vi "Task five.vi"() -> ()   [LabVIEW 2025]
uses:
  <vilib>/httpClient/POSTBuffer.vi
  <vilib>/httpClient/LabVIEWHTTPClient.lvlib
panel:
  in  "User Input":string
  in  "?":bool
  in  "Select correct word":string(combo)
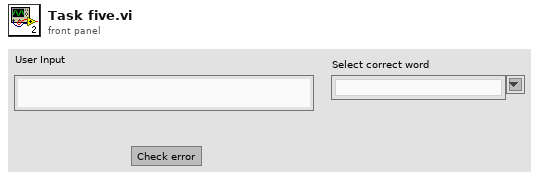
[diagram p1: front panel]
types:
  T1 = cluster{"matches":cluster{"offset":i32, "length":i32, "message":string, "replacements":cluster{"value":string}[]}[]}
  T2 = typedef "LabVIEWHTTPClient.lvlib/ClientHandle.ctl" = refnum<k1>
  T3 = cluster{"offset":i32, "length":i32, "message":string, "replacements":cluster{"value":string}[]}[]
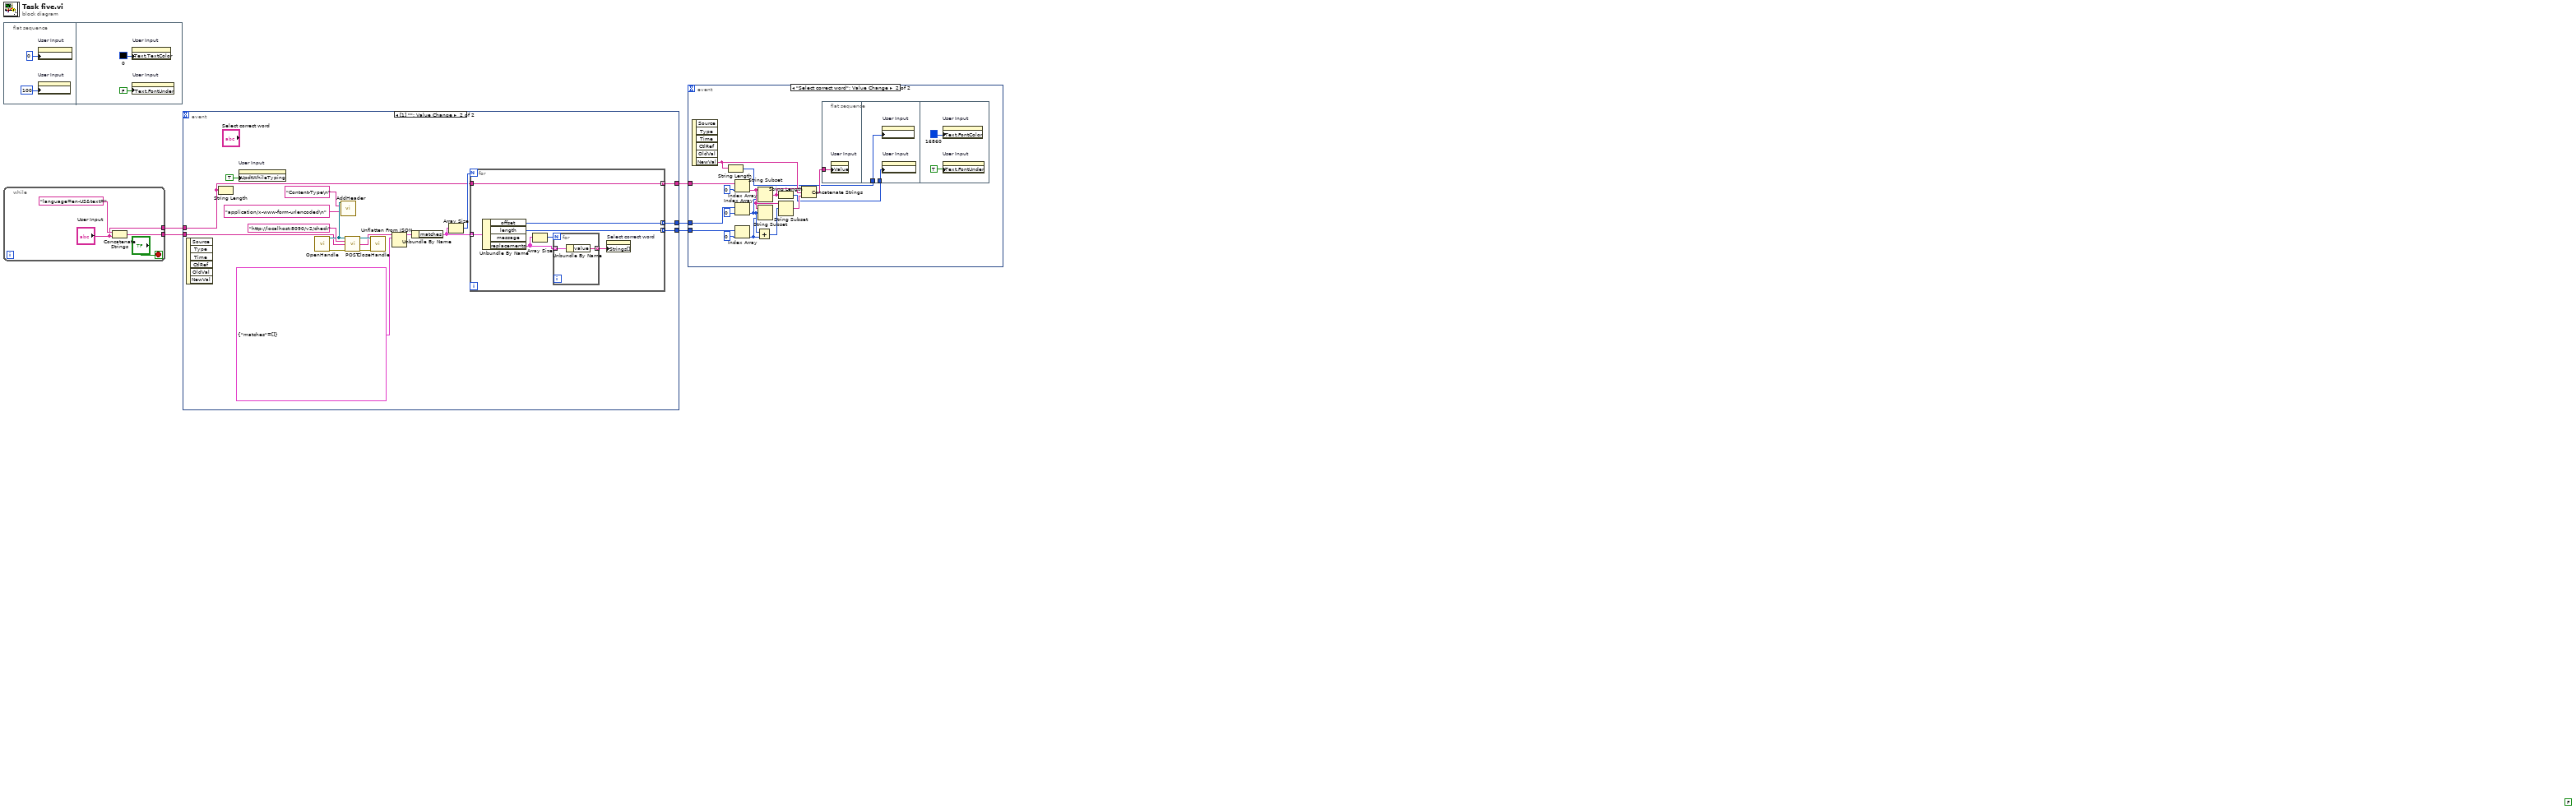
[diagram p0: block diagram]
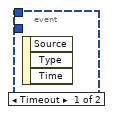
[diagram p2: hidden frame]
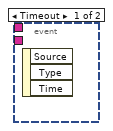
[diagram p3: hidden frame]
diagram:
  (unwired) FALSE
  n1 = flat-sequence {
    frame #0 {
      n2 = property on="User Input" class="Str"("Text.Selection Start"=0) -> ()  [unwired: 2 in, 2 out]
      n3 = property on="User Input" class="Str"("Text.Selection End"=100) -> ()  [unwired: 2 in, 2 out]
    }
    frame #1 {
      n4 = property on="User Input" class="Str"("Text.TextColor"=u32 0 ("Text.Font:Color")) -> ()  [unwired: 2 in, 2 out]
      n5 = property on="User Input" class="Str"("Text.FontUnder"=FALSE) -> ()  [unwired: 2 in, 2 out]
    }
  }
  n6 = while {
    tunnel: [w12] -> w2
    tunnel: ["User Input"] -> w1
    stop <- "?" stop-if-true
    n7 = Concatenate Strings("language=en-US&text=", "User Input") -> (w12:string)
  }
  n8 = event shown="[1] \"\": Value Change" {
    selector: _ -> [_ _]
    dyn-events: _ -> [_ _]
    timeout: _ -> [_ _]
    tunnel: w2 -> [_ w24]
    tunnel: w1 -> [_ w19]
    tunnel: [_ w17] -> w5
    tunnel: [_ w16] -> w3
    tunnel: [_ w15] -> w4
    event Timeout {
      n9 = event-data() -> ()  [unwired: 1 in, 3 out]
    }
    event Value Change {
      n10 = event-data() -> ()  [unwired: 1 in, 6 out]
      n11 = String Length(string=w19) -> ()  [unwired: 1 out]
      n12 = property on="User Input" class="Str"("UpdtWhileTyping"=TRUE ("Update While Typing?")) -> ()  [unwired: 2 in, 2 out]
      n13 = call <vilib>:"OpenHandle.vi"() -> ("client handle out"=w27:T2, "error out"=w28:errorcluster)  [unwired: 14 in]
      n14 = call <vilib>:"AddHeader.vi"("client handle"=w27, "header"="Content-Type\n", "value"="application/x-www-form-urlencoded\n") -> ()  [unwired: 11 in, 2 out]
      n15 = call-poly <vilib>:"POST.vi"("client handle"=w27, "url"="http://localhost:8090/v2/check", "buffer"=w24, "error in (no error)"=w28) -> ("client handle out"=w30:T2, "body"=w23:string, "error out"=w29:errorcluster)  [unwired: 8 in, 1 out]
      n16 = call <vilib>:"CloseHandle.vi"("client handle"=w30, "error in (no error)"=w29) -> ()  [unwired: 13 in, 1 out]
      n17 = Unflatten From JSON(JSON string=w23, type and defaults=T1 {"matches"=[]}) -> (value=w21:T1)  [unwired: 5 in, 1 out]
      n18 = Unbundle By Name(w21) -> ("matches"=w18:T3)
      n19 = Array Size(array=w18) -> (size(s)=w20:i32)
      n20 = for {
        N: w20 -> [_]
        tunnel: w18 -> [w38] mode=indexing
        tunnel: w19 -> [w32]
        tunnel: [w34] -> w17 mode=indexing
        tunnel: [w32] -> w16 mode=indexing
        tunnel: [w33] -> w15 mode=indexing
        n21 = Unbundle By Name(w38) -> ("offset"=w34:i32, "length"=w33:i32, "replacements"=w36:cluster{"value":string}[])  [unwired: 1 out]
        n22 = Array Size(array=w36) -> (size(s)=w37:i32)
        n23 = for {
          N: w37 -> [_]
          tunnel: w36 -> [w40] mode=indexing
          tunnel: [w39] -> w35 mode=indexing
          n24 = Unbundle By Name(w40) -> ("value"=w39:string)
        }
        n25 = property on="Select correct word" class="CmbBox"("Strings[]"=w35) -> ()  [unwired: 2 in, 2 out]
      }
    }
  }
  n26 = event shown="[1] \"Select correct word\": Value Change" {
    selector: _ -> [_ _]
    dyn-events: _ -> [_ _]
    timeout: _ -> [_ _]
    tunnel: w5 -> [_ w56]
    tunnel: w3 -> [_ w53]
    tunnel: w4 -> [_ w50]
    event Timeout {
      n27 = event-data() -> ()  [unwired: 1 in, 3 out]
    }
    event "Select correct word": Value Change {
      n28 = event-data() -> ("NewVal"=w42:string)  [unwired: 1 in, 5 out]
      n29 = String Length(string=w42) -> (length=w41:i32)
      n30 = Index Array(array=w53, index=0) -> (element=w52:string)
      n31 = Index Array(array=w56, index=0) -> (element=w49:i32)
      n32 = Index Array(array=w50, index=0) -> (element=w48:i32)
      n33 = Add(x=w49, y=w48) -> (x+y=w47:i32)
      n34 = String Subset(string=w52, length (rest)=w49) -> (substring=w44:string)  [unwired: 1 in]
      n35 = String Subset(string=w52, offset (0)=w49, length (rest)=w48) -> ()  [unwired: 1 out]
      n36 = String Length(string=w44) -> (length=w43:i32)
      n37 = String Subset(string=w52, offset (0)=w47) -> (substring=w46:string)  [unwired: 1 in]
      n38 = Concatenate Strings(w44, w42, w46) -> (w45:string)
      n39 = flat-sequence {
        tunnel: w45 -> [w57]
        tunnel: w43 -> [w59]
        tunnel: w41 -> [w58]
        frame #0 {
          n40 = property on="User Input" class="Str"("Value"=w57) -> ()  [unwired: 2 in, 2 out]
        }
        frame #1 {
          n41 = property on="User Input" class="Str"("Text.Selection End"=w58) -> ()  [unwired: 2 in, 2 out]
          n42 = property on="User Input" class="Str"("Text.Selection Start"=w59) -> ()  [unwired: 2 in, 2 out]
        }
        frame #2 {
          n43 = property on="User Input" class="Str"("Text.FontColor"=u32 16860 ("Text.Font:Color")) -> ()  [unwired: 2 in, 2 out]
          n44 = property on="User Input" class="Str"("Text.FontUnder"=TRUE) -> ()  [unwired: 2 in, 2 out]
        }
      }
    }
  }
